vi "Format Array to String.vi"(11 "subarray":string[](array[string])) -> (3 "String":string)   [LabVIEW 2020]
panel:
  out "Array":string[](array[string])
  out "length":i32
  # "8200013$"
  # "%%%%%%%%"
  # "%%%%%%%%%"
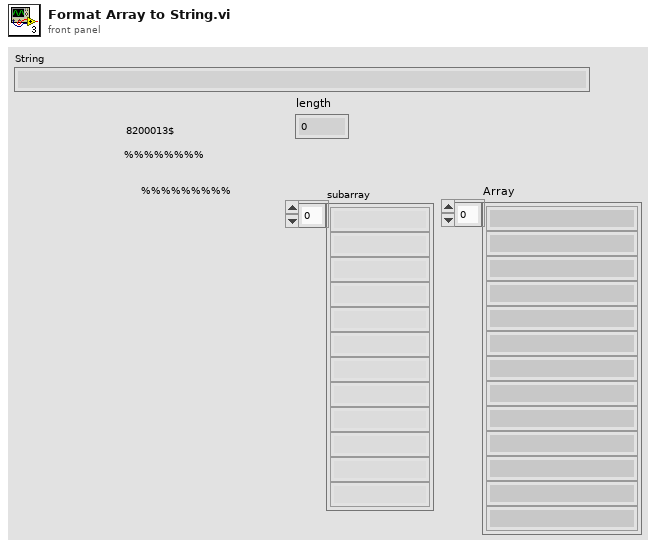
[diagram p1: front panel]
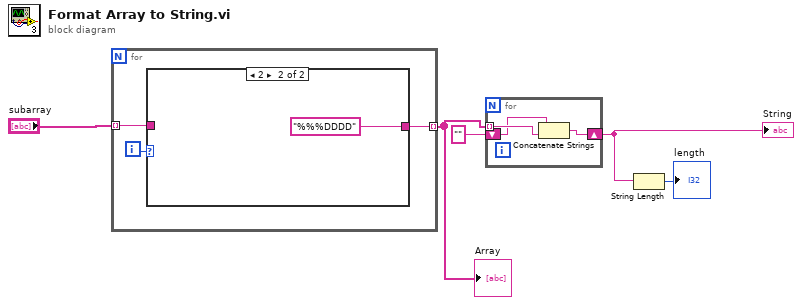
[diagram p0: block diagram]
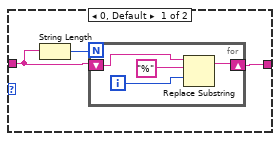
[diagram p2: hidden frame]
diagram:
  n1 = for {
    tunnel: "subarray" -> [w8] mode=indexing
    tunnel: [w7] -> w4 mode=indexing
    i -> [w6]
    n2 = case shown="2" w6 {
      tunnel: w8 -> [w10 _]
      tunnel: [w9 "%%%DDDD" ("date/time string")] -> w7
      frame 0, Default {
        n3 = String Length(string=w10) -> (length=w11:i32)
        n4 = for {
          N: w11 -> [_]
          shift-right: [w13] -> w9
          shift-left: w10 -> [w14]
          i -> [w12]
          n5 = Replace Substring(3:w12, 4:"%" ("substring (\"\")"), 5:w14) -> (1:w13:string)  [unwired: 1 in, 1 out]
        }
      }
      frame 2 {
      }
    }
  }
  "Array" <- w4
  n6 = for {
    tunnel: w4 -> [w18] mode=indexing
    shift-right: [w19] -> w1
    shift-left: "" -> [w17]
    n7 = Concatenate Strings(w17, w18) -> (w19:string)
  }
  "String" <- w1
  n8 = String Length(string=w1) -> (length=→"length":i32)
